vi "[Template]_Static Read.vi"(8 "error in (no error)":errorcluster, 9 "Default":T1, 11 "Tag Name":string) -> (0 "error out":errorcluster, 1 "Data":T1)   [LabVIEW 2010]
doc: "This VI will read the data associated with a single tag. This VI will only look up the tag index on the first call, or if the look-up resulted in an error. This VI has higher performance than the normal read function thanks to the removal of the name check."
uses:
  [Template]_Datatype.ctl
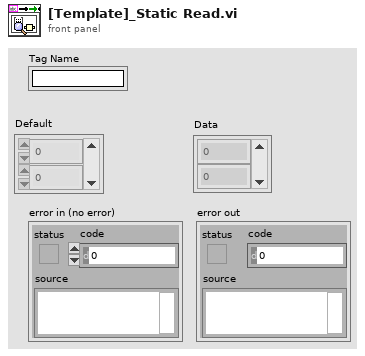
[diagram p1: front panel]
types:
  T1 = typedef "[Template]_Datatype.ctl" = i32[]
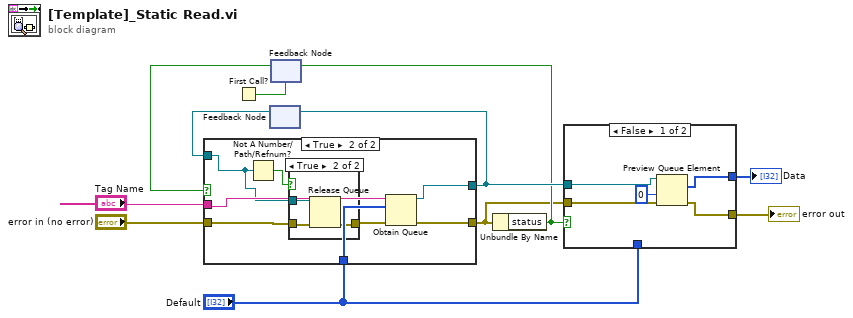
[diagram p0: block diagram]
diagram:
  n1 = First Call?() -> (First Call?: T/F=w6:bool)
  n2 = feedback #1() -> (w10:refnum<queue>)  [unwired: 1 in]
  n3 = feedback #2(w6) -> (w5:bool)
  n4 = case shown="True" w5 {
    tunnel: [w13 w19] -> w2
    tunnel: "error in (no error)" -> [w13 w15]
    tunnel: [w12 w20] -> w9
    tunnel: w10 -> [w12 w16]
    tunnel: "Tag Name" -> [_ w18]
    tunnel: "Default" -> [_ w21]
    frame False {
    }
    frame True {
      n5 = Not A Number/Path/Refnum?(number/path/refnum=w16) -> (NaN/Path/Refnum?=w17:bool)
      n6 = case shown="True" w17 {
        tunnel: w15 -> [w22 w24]
        tunnel: [w22 w25] -> w14
        tunnel: w16 -> [_ w23]
        frame False {
        }
        frame True {
          n7 = Release Queue(queue=w23, error in (no error)=w24) -> (error out=w25:errorcluster)  [unwired: 1 in, 2 out]
        }
      }
      n8 = Obtain Queue(name (unnamed)=w18, element data type=w21, error in (no error)=w14) -> (queue out=w20:refnum<queue>, error out=w19:errorcluster)  [unwired: 2 in, 1 out]
    }
  }
  n9 = feedback-in #1(w9) -> ()
  n10 = Unbundle By Name(w2) -> ("status"=w7:bool)
  n11 = feedback-in #2(w7) -> ()
  n12 = case shown="False" w7 {
    tunnel: w9 -> [w30 _]
    tunnel: "Default" -> [_ w32]
    tunnel: [w27 w32] -> w4
    tunnel: w2 -> [w29 w31]
    tunnel: [w28 w31] -> w1
    frame False {
      n13 = Preview Queue Element(queue=w30, timeout in ms (-1)=0, error in (no error)=w29) -> (element=w27:T1, error out=w28:errorcluster)  [unwired: 2 out]
    }
    frame True {
    }
  }
  "Data" <- w4
  "error out" <- w1
